vi "isAsserted.vi"(11 "Leaf.Properties.Assert":refnum<class "Leaf.Properties.Assert.lvclass">) -> (1 "Skipped":bool, 2 "Asserted":bool, 3 "Leaf.Properties.Assert":refnum<class "Leaf.Properties.Assert.lvclass">)   [LabVIEW 2021, in "Banana.Caraya.lvlib" / "Leaf.Properties.Assert.lvclass"]
uses:
  Leaf.Properties.Assert.lvclass
  <vilib>/addons/_JKI Toolkits/Caraya/classes/Properties.Assert/Properties.Assert.lvclass/Properties.Assert.ctl
  Leaf.Properties.Assert.lvclass/Leaf.Properties.Assert.ctl
  <vilib>/addons/_JKI Toolkits/Caraya/classes/Properties.Assert/Properties.Assert.lvclass
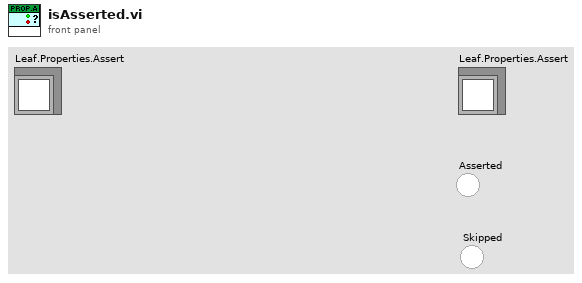
[diagram p1: front panel]
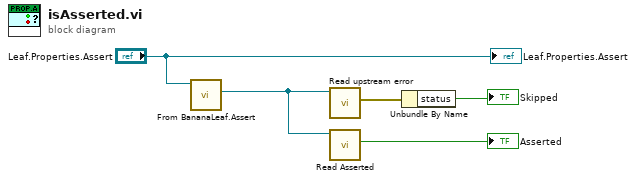
[diagram p0: block diagram]
diagram:
  n1 = call "From BananaLeaf.Assert.vi"("Leaf.Properties.Assert"="Leaf.Properties.Assert") -> ("Properties.Assert"=w1:refnum<class "Properties.Assert.lvclass">)  [unwired: 10 in]
  n2 = call <vilib>:"Read upstream error.vi"("Properties.Assert in"=w1) -> ("upstream-error"=w4:errorcluster)  [unwired: 9 in, 1 out]
  n3 = call <vilib>:"Read Asserted.vi"("Properties.Assert in"=w1) -> ("Asserted"=→"Asserted":bool)  [unwired: 9 in, 1 out]
  n4 = Unbundle By Name(w4) -> ("status"=→"Skipped":bool)
  "Leaf.Properties.Assert" <- "Leaf.Properties.Assert"
